vi "RemoveNodes.vi"(6 "RemoveSearch":T1={"LLSearch"=refnum, "length"=1}, 8 "error in (no error)":errorcluster, 9 "position":T2, 11 "LinkedList in":refnum<class "LinkedList.lvclass">) -> (0 "error out":errorcluster, 1 "ignored":bool, 2 "RemovedNode":refnum<data-value>, 3 "LinkedList out":refnum<class "LinkedList.lvclass">)   [LabVIEW 2009, in "LinkedList.lvclass"]
uses:
  LinkedList.lvclass
  position.ctl
  LLNode/LLNode.lvclass
  RemoveSearch.ctl
  LLSearch/LLSearch.lvclass
  Node/Node.lvclass
  Structure/Structure.lvclass
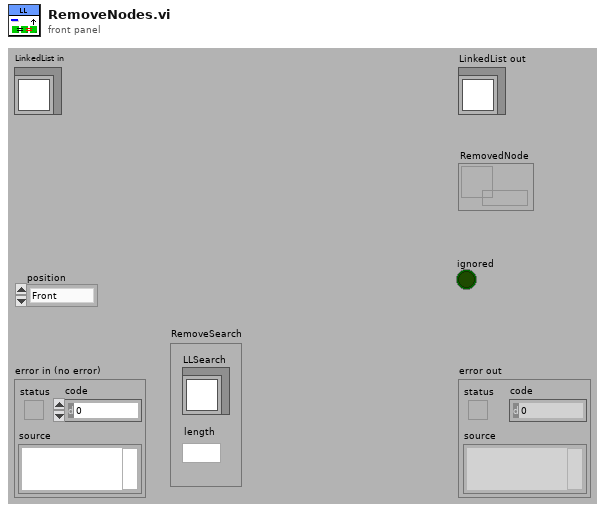
[diagram p1: front panel]
types:
  T1 = typedef "LinkedList.lvclass/RemoveSearch.ctl" = cluster{"LLSearch":refnum<class "LLSearch.lvclass">, "length":u32}
  T2 = typedef "LinkedList.lvclass/position.ctl" = enum16{"Front", "Back", "Search"}
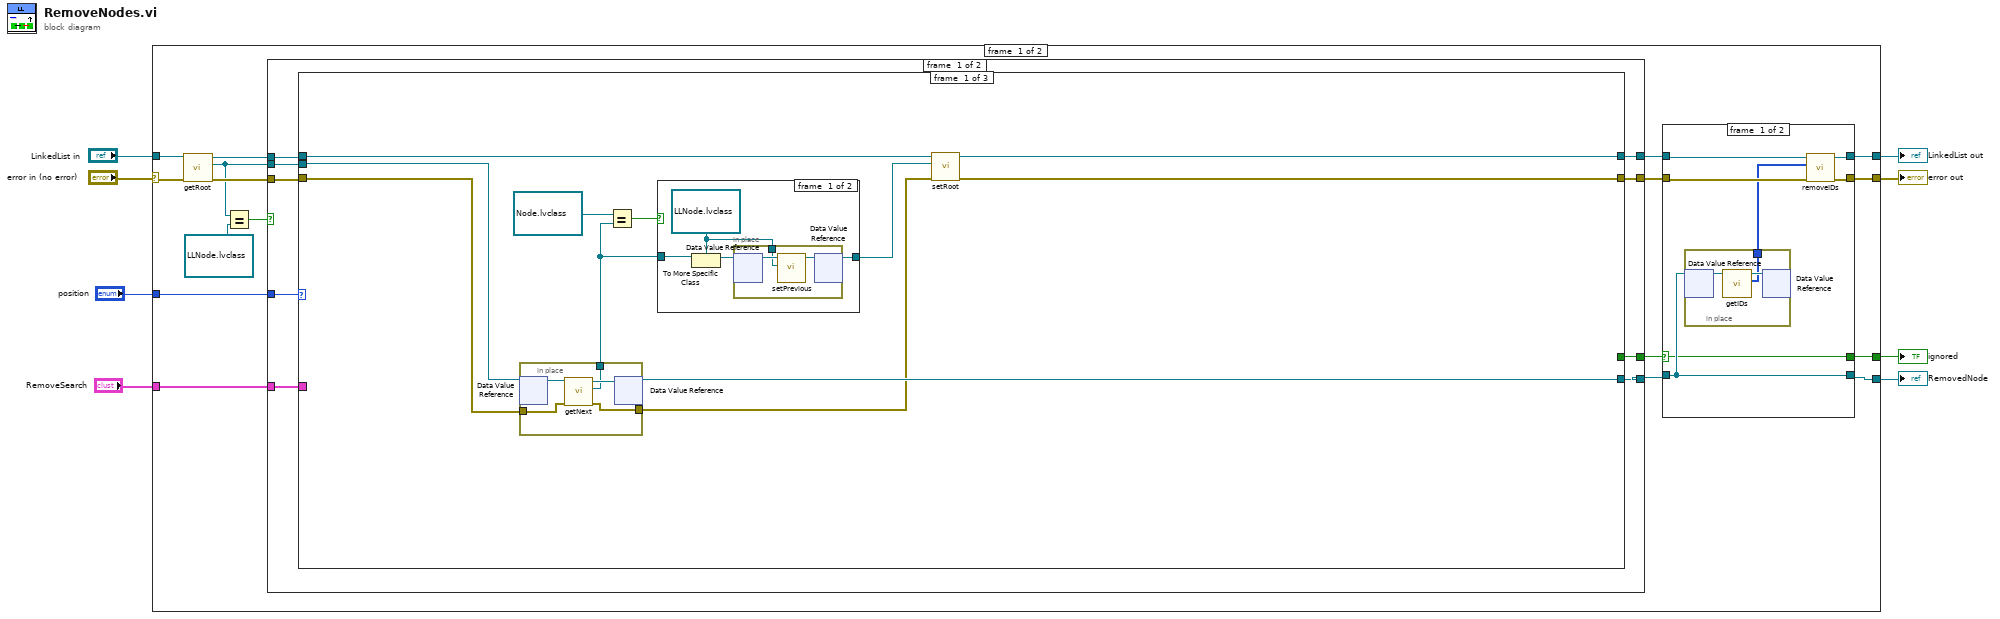
[diagram p0: block diagram]
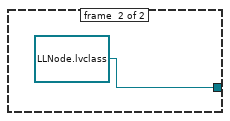
[diagram p3: hidden frame]
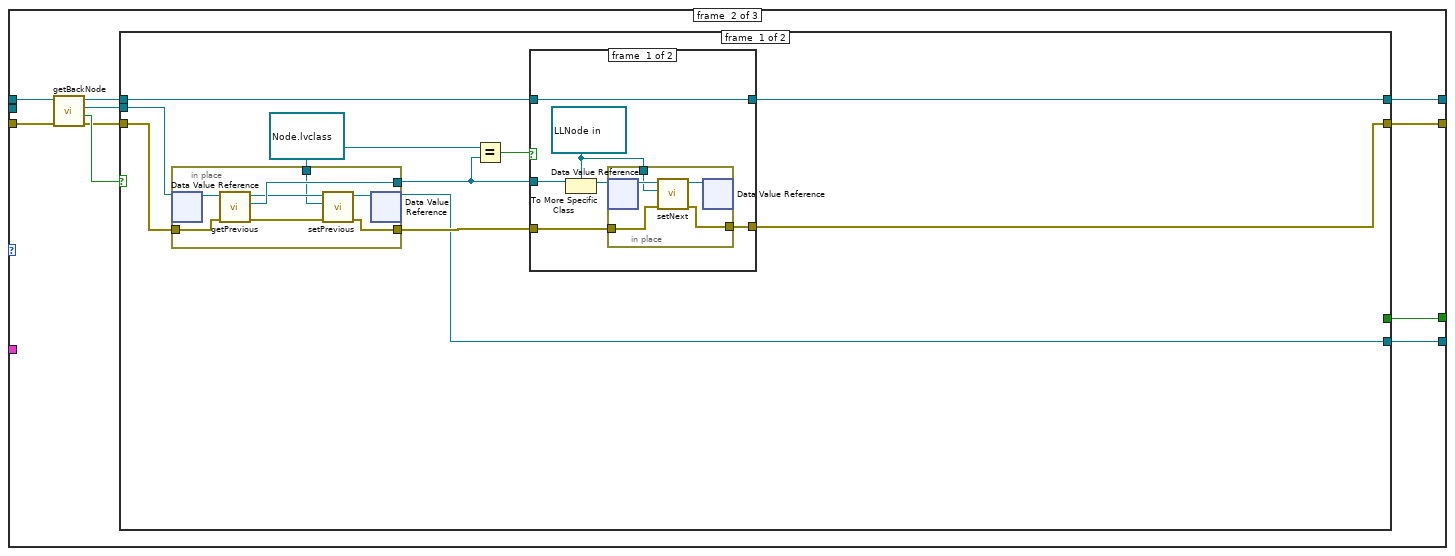
[diagram p4: hidden frame]
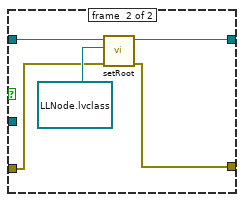
[diagram p5: hidden frame]
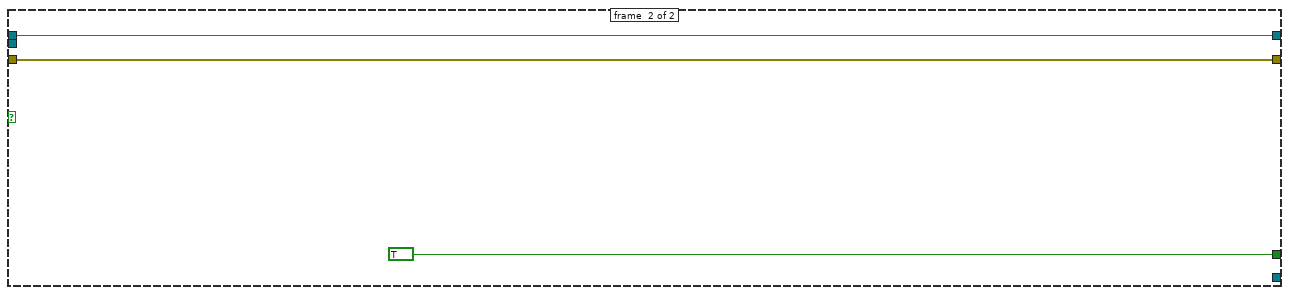
[diagram p6: hidden frame]
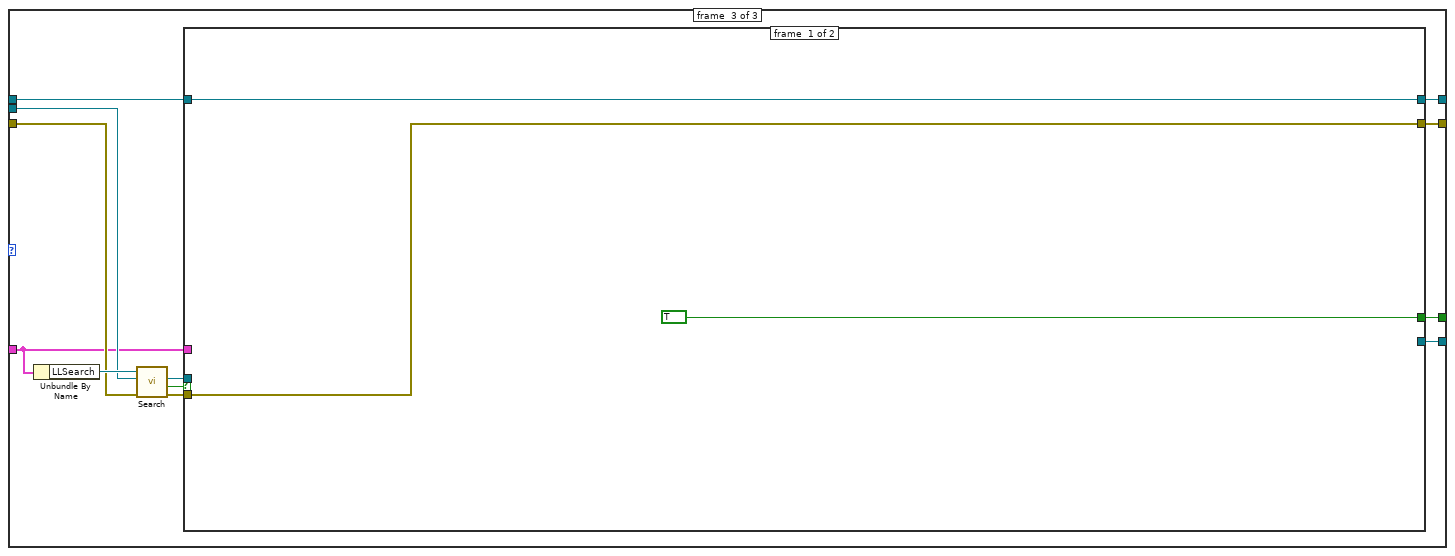
[diagram p7: hidden frame]
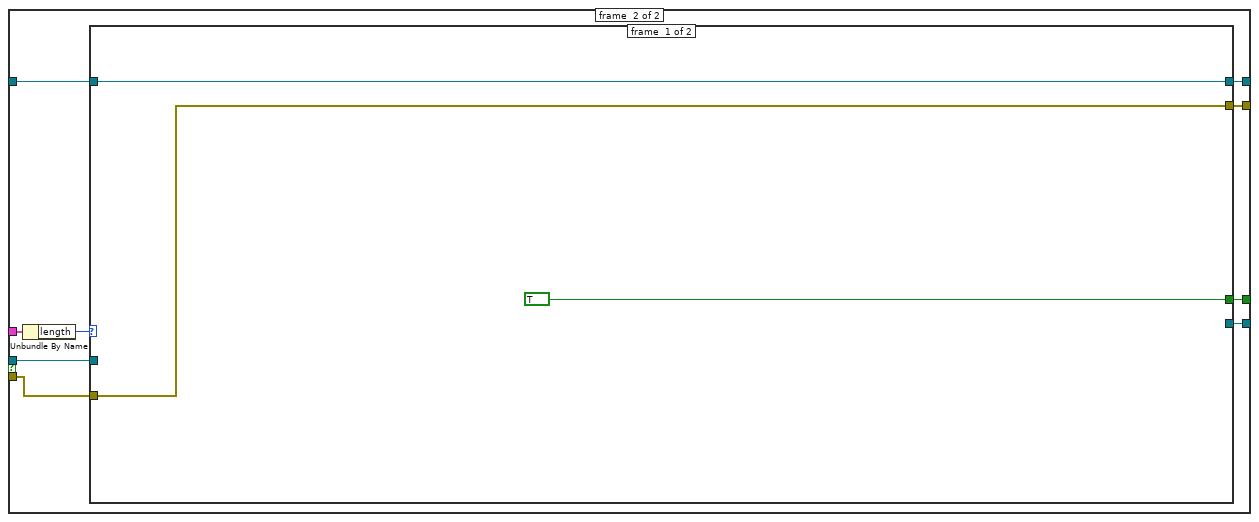
[diagram p8: hidden frame]
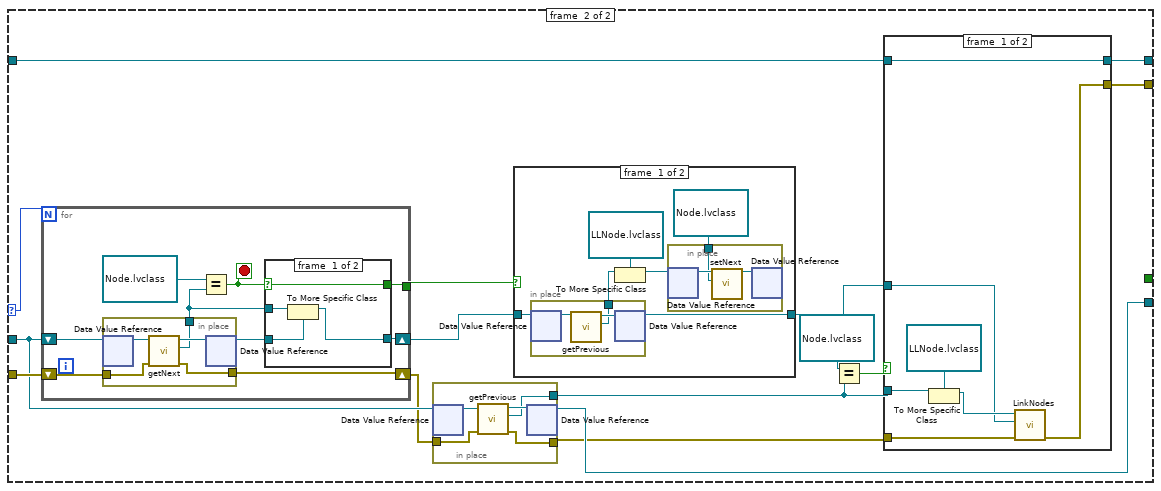
[diagram p9: hidden frame]
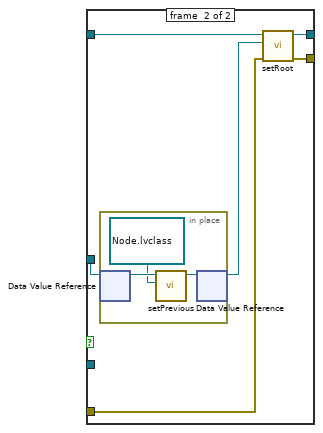
[diagram p11: hidden frame]
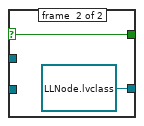
[diagram p12: hidden frame]
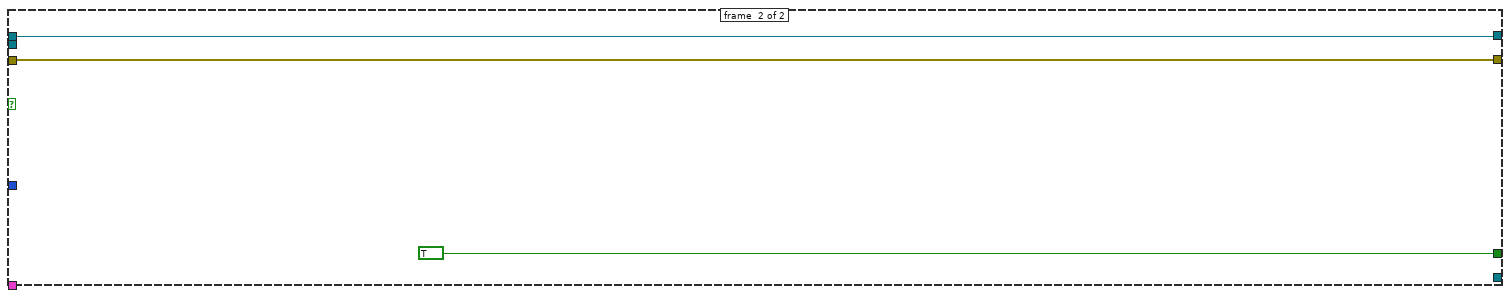
[diagram p13: hidden frame]
diagram:
  n1 = case shown="No Error" "error in (no error)" {
    selector: "error in (no error)" -> [w22 w220]
    tunnel: [w11 w220] -> w7
    tunnel: [w12 w219] -> w5
    tunnel: "LinkedList in" -> [w23 w219]
    tunnel: "position" -> [w25 _]
    tunnel: "RemoveSearch" -> [w24 _]
    tunnel: [w9 _] -> w2
    tunnel: [w10 _] -> w1
    frame #0 {
      n2 = call "getRoot.vi"("error in (no error)"=w22, "LinkedList in"=w23) -> ("error out"=w21:errorcluster, "Root"=w17:refnum<data-value>, "LinkedList out"=w20:refnum<class "LinkedList.lvclass">)  [unwired: 7 in]
      n3 = Equal?(x=w17, y=refnum<data-value> refnum) -> (x = y?=w18:bool)
      n4 = case shown="False" w18 {
        tunnel: w25 -> [w48 _]
        tunnel: w24 -> [w47 _]
        tunnel: [w46 TRUE] -> w16
        tunnel: [w45 w218] -> w14
        tunnel: [w44 w217] -> w13
        tunnel: [w43 _] -> w15
        tunnel: w21 -> [w42 w217]
        tunnel: w20 -> [w41 w218]
        tunnel: w17 -> [w40 _]
        frame #0 {
          n5 = case shown="\"Search\"" w48 {
            tunnel: w41 -> [w50 w82 w129]
            tunnel: w47 -> [_ _ w123]
            tunnel: [_ w73 w124] -> w46
            tunnel: w42 -> [w49 w79 w126]
            tunnel: [w59 w76 w122] -> w45
            tunnel: [w58 w75 w121] -> w44
            tunnel: [w57 w74 w120] -> w43
            tunnel: w40 -> [w51 _ w130]
            frame #0 {
              n6 = in-place {
                in-place-border: w49 -> [w71]
                in-place-border: [w69] -> w52
                in-place-border: [w68] -> w54
                n7 = in-place-dvr #1(w51) -> (w72:refnum<class "LLNode.lvclass">)  [unwired: 1 out]
                n8 = call "getNext.vi"("error in (no error)"=w71, "LLNode in"=w72) -> ("error out"=w69:errorcluster, "next"=w68:refnum<data-value>, "LLNode out"=w70:refnum<class "LLNode.lvclass">)  [unwired: 7 in]
                n9 = in-place-dvr #1(w70) -> (w57:refnum<data-value>)  [unwired: 1 out]
              }
              n10 = Equal?(x=refnum<data-value> refnum, y=w54) -> (x = y?=w55:bool)
              n11 = case shown="False" w55 {
                tunnel: w54 -> [w63 _]
                tunnel: [w61 refnum<data-value> refnum ("Root")] -> w53
                frame #0 {
                  w60 = refnum<data-value> refnum ("y")
                  n12 = To More Specific Class(target class=w60, reference=w63) -> (specific class reference=w62:refnum<data-value>)  [unwired: 1 in, 1 out]
                  n13 = in-place {
                    in-place-border: w60 -> [w64]
                    n14 = in-place-dvr #2(w62) -> (w66:refnum<class "LLNode.lvclass">)  [unwired: 1 out]
                    n15 = call "setPrevious.vi"("previous"=w64, "LLNode in"=w66) -> ("LLNode out"=w65:refnum<class "LLNode.lvclass">)  [unwired: 8 in, 1 out]
                    n16 = in-place-dvr #2(w65) -> (w61:refnum<data-value>)  [unwired: 1 out]
                  }
                }
                frame #1 {
                }
              }
              n17 = call "setRoot.vi"("error in (no error)"=w52, "Root"=w53, "LinkedList in"=w50) -> ("error out"=w58:errorcluster, "LinkedList out"=w59:refnum<class "LinkedList.lvclass">)  [unwired: 7 in]
            }
            frame #1 {
              n18 = call "getBackNode.vi"("error in (no error)"=w79, "LinkedList in"=w82) -> ("error out"=w77:errorcluster, "ignored"=w81:bool, "BackNode"=w78:refnum<data-value>, "LinkedList out"=w80:refnum<class "LinkedList.lvclass">)  [unwired: 6 in]
              n19 = case shown="False" w81 {
                tunnel: w80 -> [w90 w118]
                tunnel: w78 -> [w92 _]
                tunnel: w77 -> [w91 w117]
                tunnel: [w86 w118] -> w76
                tunnel: [w85 w117] -> w75
                tunnel: [w84 _] -> w74
                tunnel: [_ TRUE] -> w73
                frame #0 {
                  w83 = refnum<data-value> refnum ("previous")
                  n20 = in-place {
                    in-place-border: w91 -> [w110]
                    in-place-border: [w112] -> w87
                    in-place-border: [w116] -> w88
                    in-place-border: w83 -> [w109]
                    n21 = in-place-dvr #3(w92) -> (w115:refnum<class "LLNode.lvclass">)  [unwired: 1 out]
                    n22 = call "getPrevious.vi"("error in (no error)"=w110, "LLNode in"=w115) -> ("error out"=w111:errorcluster, "previous"=w116:refnum<data-value>, "LLNode out"=w114:refnum<class "LLNode.lvclass">)  [unwired: 7 in]
                    n23 = call "setPrevious.vi"("error in (no error)"=w111, "previous"=w109, "LLNode in"=w114) -> ("error out"=w112:errorcluster, "LLNode out"=w113:refnum<class "LLNode.lvclass">)  [unwired: 7 in]
                    n24 = in-place-dvr #3(w113) -> (w84:refnum<data-value>)  [unwired: 1 out]
                  }
                  n25 = Equal?(x=w83, y=w88) -> (x = y?=w89:bool)
                  n26 = case shown="True" w89 {
                    tunnel: w90 -> [w97 w108]
                    tunnel: w88 -> [w98 _]
                    tunnel: w87 -> [w94 w105]
                    tunnel: [w97 w106] -> w86
                    tunnel: [w93 w104] -> w85
                    frame #0 {
                      w95 = refnum<data-value> refnum ("BackNode")
                      n27 = To More Specific Class(target class=w95, reference=w98) -> (specific class reference=w96:refnum<data-value>)  [unwired: 1 in, 1 out]
                      n28 = in-place {
                        in-place-border: w95 -> [w101]
                        in-place-border: w94 -> [w100]
                        in-place-border: [w99] -> w93
                        n29 = in-place-dvr #4(w96) -> (w103:refnum<class "LLNode.lvclass">)  [unwired: 1 out]
                        n30 = call "setNext.vi"("error in (no error)"=w100, "next"=w101, "LLNode in"=w103) -> ("error out"=w99:errorcluster, "LLNode out"=w102:refnum<class "LLNode.lvclass">)  [unwired: 7 in]
                        n31 = in-place-dvr #4(w102) -> ()  [unwired: 2 out]
                      }
                    }
                    frame #1 {
                      n32 = call "setRoot.vi"("error in (no error)"=w105, "Root"=refnum<data-value> refnum, "LinkedList in"=w108) -> ("error out"=w104:errorcluster, "LinkedList out"=w106:refnum<class "LinkedList.lvclass">)  [unwired: 7 in]
                    }
                  }
                }
                frame #1 {
                }
              }
            }
            frame #2 {
              n33 = Unbundle By Name(w123) -> ("LLSearch"=w131:refnum<class "LLSearch.lvclass">)
              n34 = call "Search.vi"("error in (no error)"=w126, "LLNode in"=w130, "LLSearch in"=w131) -> ("error out"=w125:errorcluster, "found"=w128:bool, "LLNode out"=w127:refnum<data-value>)  [unwired: 5 in, 1 out]
              n35 = case shown="True" w128 {
                tunnel: w129 -> [w133 w138]
                tunnel: w127 -> [_ w142]
                tunnel: w125 -> [w132 w141]
                tunnel: [TRUE w139] -> w124
                tunnel: w123 -> [_ w143]
                tunnel: [w133 w137] -> w122
                tunnel: [w132 w136] -> w121
                tunnel: [_ w135] -> w120
                frame #0 {
                }
                frame #1 {
                  n36 = Unbundle By Name(w143) -> ("length"=w140:u32)
                  n37 = case shown="Default" w140 {
                    selector: w140 -> [_ w160]
                    tunnel: w142 -> [_ w159]
                    tunnel: w141 -> [w144 w161]
                    tunnel: [TRUE _] -> w139
                    tunnel: w138 -> [w145 w158]
                    tunnel: [w145 w153] -> w137
                    tunnel: [w144 w152] -> w136
                    tunnel: [_ w151] -> w135
                    frame #0 {
                    }
                    frame #1 {
                      n38 = for {
                        N: w160 -> [_]
                        shift-right: [w199] -> w148
                        shift-left: w159 -> [w202]
                        shift-right: [w197] -> w156
                        shift-left: w161 -> [w204]
                        tunnel: [w196] -> w149
                        stop <- w201 stop-if-true
                        n39 = in-place {
                          in-place-border: w204 -> [w213]
                          in-place-border: [w212] -> w198
                          in-place-border: [w211] -> w197
                          n40 = in-place-dvr #5(w202) -> (w215:refnum<class "LLNode.lvclass">)  [unwired: 1 out]
                          n41 = call "getNext.vi"("error in (no error)"=w213, "LLNode in"=w215) -> ("error out"=w211:errorcluster, "next"=w212:refnum<data-value>, "LLNode out"=w214:refnum<class "LLNode.lvclass">)  [unwired: 7 in]
                          n42 = in-place-dvr #5(w214) -> (w200:refnum<data-value>)  [unwired: 1 out]
                        }
                        n43 = Equal?(x=refnum<data-value> refnum, y=w198) -> (x = y?=w201:bool)
                        n44 = case shown="True" w201 {
                          selector: w201 -> [w205 w209]
                          tunnel: w200 -> [w207 _]
                          tunnel: [w206 refnum<data-value> refnum ("LLNode out")] -> w199
                          tunnel: w198 -> [w208 _]
                          tunnel: [w205 w209] -> w196
                          frame #0 {
                            n45 = To More Specific Class(target class=w207, reference=w208) -> (specific class reference=w206:refnum<data-value>)  [unwired: 1 in, 1 out]
                          }
                          frame #1 {
                          }
                        }
                      }
                      n46 = in-place {
                        in-place-border: [w193] -> w154
                        in-place-border: w156 -> [w192]
                        in-place-border: [w191] -> w150
                        n47 = in-place-dvr #6(w159) -> (w195:refnum<class "LLNode.lvclass">)  [unwired: 1 out]
                        n48 = call "getPrevious.vi"("error in (no error)"=w192, "LLNode in"=w195) -> ("error out"=w191:errorcluster, "previous"=w193:refnum<data-value>, "LLNode out"=w194:refnum<class "LLNode.lvclass">)  [unwired: 7 in]
                        n49 = in-place-dvr #6(w194) -> (w151:refnum<data-value>)  [unwired: 1 out]
                      }
                      n50 = case shown="False" w149 {
                        tunnel: w148 -> [w167 w174]
                        tunnel: [w166 w174] -> w147
                        frame #0 {
                          n51 = in-place {
                            in-place-border: [w171] -> w165
                            n52 = in-place-dvr #7(w167) -> (w173:refnum<class "LLNode.lvclass">)  [unwired: 1 out]
                            n53 = call "getPrevious.vi"("LLNode in"=w173) -> ("previous"=w171:refnum<data-value>, "LLNode out"=w172:refnum<class "LLNode.lvclass">)  [unwired: 8 in, 1 out]
                            n54 = in-place-dvr #7(w172) -> (w166:refnum<data-value>)  [unwired: 1 out]
                          }
                          n55 = To More Specific Class(target class=refnum<data-value> refnum ("LLNode out"), reference=w165) -> (specific class reference=w163:refnum<data-value>)  [unwired: 1 in, 1 out]
                          n56 = in-place {
                            in-place-border: refnum<data-value> refnum ("x") -> [w168]
                            n57 = in-place-dvr #8(w163) -> (w170:refnum<class "LLNode.lvclass">)  [unwired: 1 out]
                            n58 = call "setNext.vi"("next"=w168, "LLNode in"=w170) -> ("LLNode out"=w169:refnum<class "LLNode.lvclass">)  [unwired: 8 in, 1 out]
                            n59 = in-place-dvr #8(w169) -> ()  [unwired: 2 out]
                          }
                        }
                        frame #1 {
                        }
                      }
                      n60 = Equal?(x=refnum<data-value> refnum, y=w154) -> (x = y?=w157:bool)
                      n61 = case shown="False" w157 {
                        tunnel: w158 -> [w181 w186]
                        tunnel: w147 -> [w176 w187]
                        tunnel: w150 -> [w178 w184]
                        tunnel: w154 -> [w180 _]
                        tunnel: [w181 w183] -> w153
                        tunnel: [w175 w182] -> w152
                        frame #0 {
                          n62 = To More Specific Class(target class=refnum<data-value> refnum ("LLNode out"), reference=w180) -> (specific class reference=w177:refnum<data-value>)  [unwired: 1 in, 1 out]
                          n63 = call "LinkNodes.vi"("error in (no error)"=w178, "NextNode in"=w176, "PreviousNode in"=w177) -> ("error out"=w175:errorcluster)  [unwired: 6 in, 2 out]
                        }
                        frame #1 {
                          n64 = in-place {
                            n65 = in-place-dvr #9(w187) -> (w190:refnum<class "LLNode.lvclass">)  [unwired: 1 out]
                            n66 = call "setPrevious.vi"("previous"=refnum<data-value> refnum, "LLNode in"=w190) -> ("LLNode out"=w188:refnum<class "LLNode.lvclass">)  [unwired: 8 in, 1 out]
                            n67 = in-place-dvr #9(w188) -> (w185:refnum<data-value>)  [unwired: 1 out]
                          }
                          n68 = call "setRoot.vi"("error in (no error)"=w184, "Root"=w185, "LinkedList in"=w186) -> ("error out"=w182:errorcluster, "LinkedList out"=w183:refnum<class "LinkedList.lvclass">)  [unwired: 7 in]
                        }
                      }
                    }
                  }
                }
              }
            }
          }
        }
        frame #1 {
        }
      }
      n69 = case shown="False" w16 {
        selector: w16 -> [w27 w39]
        tunnel: w15 -> [w32 w38]
        tunnel: w14 -> [w29 w37]
        tunnel: w13 -> [w28 w36]
        tunnel: [w31 w37] -> w12
        tunnel: [w30 w36] -> w11
        tunnel: [w32 w38] -> w10
        tunnel: [w27 w39] -> w9
        frame #0 {
          n70 = in-place {
            in-place-border: [w33] -> w26
            n71 = in-place-dvr #10(w32) -> (w35:refnum<class "LLNode.lvclass">)  [unwired: 1 out]
            n72 = call "getIDs.vi"("LLNode in"=w35) -> ("IDs"=w33:u32[], "LLNode out"=w34:refnum<class "LLNode.lvclass">)  [unwired: 8 in, 1 out]
            n73 = in-place-dvr #10(w34) -> ()  [unwired: 2 out]
          }
          n74 = call "removeIDs.vi"("error in (no error)"=w28, "IDs"=w26, "Structure in"=w29) -> ("error out"=w30:errorcluster, "Structure out"=w31:refnum<class "LinkedList.lvclass">)  [unwired: 7 in]
        }
        frame #1 {
        }
      }
    }
    frame #1 {
    }
  }
  "error out" <- w7
  "LinkedList out" <- w5
  "RemovedNode" <- w1
  "ignored" <- w2
